vi "Panel Init Dry Meter.vi"() -> (2 "Init Dry Meter Reading Out":string)   [LabVIEW 2009]
panel:
  in  "Enter Dry Meter Reading":string
  in  "stop":bool
  # "(xxx.xxx)"
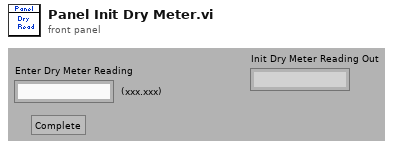
[diagram p1: front panel]
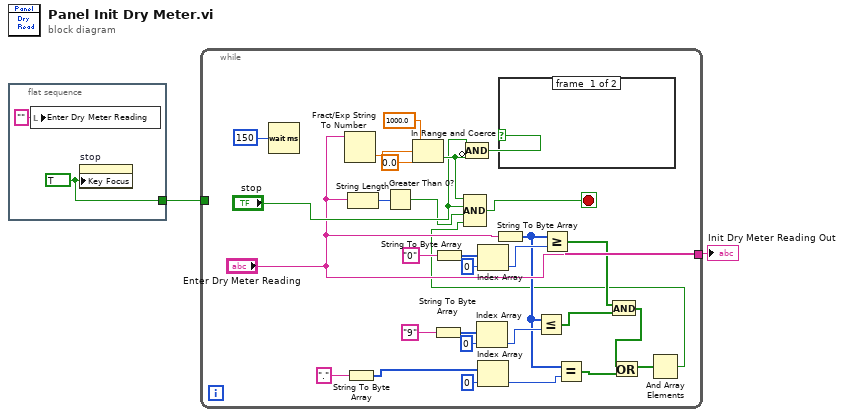
[diagram p0: block diagram]
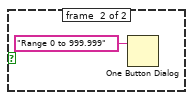
[diagram p2: hidden frame]
diagram:
  n1 = flat-sequence {
    tunnel: [w4] -> w1
    frame #0 {
      w4 = TRUE ("Key Focus")
      n2 = local write "Enter Dry Meter Reading"("" ("Enter Dry Meter Reading")) -> ()
      n3 = property on="stop" class="Bool"("Key Focus"=w4) -> ()  [unwired: 2 in, 2 out]
    }
  }
  n4 = while {
    tunnel: ["Enter Dry Meter Reading"] -> w2
    tunnel: w1 -> [_]
    stop <- w30 stop-if-true
    n5 = Wait (ms)(milliseconds to wait=u32 150) -> ()  [unwired: 1 out]
    n6 = Fract/Exp String To Number(string="Enter Dry Meter Reading") -> (number=w33:dbl)  [unwired: 3 in, 1 out]
    n7 = String To Byte Array(string=".") -> (unsigned byte array=w13:u8[])
    n8 = String Length(string="Enter Dry Meter Reading") -> (length=w26:i32)
    n9 = Greater Than 0?(x=w26) -> (x > 0?=w25:bool)
    n10 = In Range and Coerce(upper limit=1000.0, x=w33, lower limit=0.0) -> (In Range?=w29:bool)  [unwired: 1 out]
    n11 = String To Byte Array(string="9") -> (unsigned byte array=w17:u8[])
    n12 = String To Byte Array(string="0") -> (unsigned byte array=w21:u8[])
    n13 = Compound Arithmetic op=AND("stop", invert w29) -> (w28:bool)
    n14 = Index Array(array=w17, index=0) -> (element=w15:u8)
    n15 = Index Array(array=w21, index=0) -> (element=w19:u8)
    n16 = Index Array(array=w13, index=0) -> (element=w11:u8)
    n17 = String To Byte Array(string="Enter Dry Meter Reading") -> (unsigned byte array=w12:u8[])
    n18 = case shown="False" w28 {
      frame #0 {
      }
      frame #1 {
        n19 = One Button Dialog(message="Range 0 to 999.999") -> ()  [unwired: 1 in, 1 out]
      }
    }
    n20 = Less Or Equal?(x=w12, y=w15) -> (x <= y?=w10:bool[])
    n21 = Greater Or Equal?(x=w12, y=w19) -> (x >= y?=w9:bool[])
    n22 = Equal?(x=w12, y=w11) -> (x = y?=w8:bool[])
    n23 = And(x=w9, y=w10) -> (x .and. y?=w7:bool[])
    n24 = Or(x=w7, y=w8) -> (x .or. y?=w6:bool[])
    n25 = And Array Elements(Boolean array=w6) -> (logical AND=w5:bool)
    n26 = Compound Arithmetic op=AND(w29, "stop", w25, w5) -> (w30:bool)
  }
  "Init Dry Meter Reading Out" <- w2
